vi "Acquire Data (Simulated).vi"(0 "# of points":i32) -> (1 "data":sgl[](array[numeric]) format="%0.2f", 2 "time":string)   [LabVIEW 2011]
doc: "Generates simulated waveforms given the size n points of the wave"
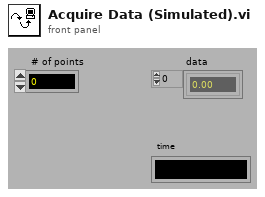
[diagram p1: front panel]
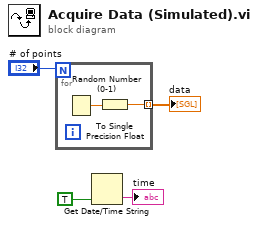
[diagram p0: block diagram]
diagram:
  n1 = for {
    N: "# of points" -> [_]
    tunnel: [w5] -> w2 mode=indexing
    n2 = Random Number (0-1)() -> (number: 0 to 1=w6:dbl)
    n3 = To Single Precision Float(number=w6) -> (single precision float=w5:sgl)
  }
  "data" <- w2
  n4 = Get Date/Time String(want seconds? (F)=TRUE) -> (time string=→"time":string)  [unwired: 3 out]
